vi "TCCII.vi"() -> ()   [LabVIEW 2019]
uses:
  <vilib>/Utility/NIReport.llb/Report Type.ctl
  <vilib>/Utility/NIReport.llb/image depth.ctl
  <vilib>/Instr/_visa.llb/VISA Configure Serial Port (Instr).vi
  <vilib>/Utility/NIReport.llb/Append Report Text (str wrap).vi
  <vilib>/printing/OpenHTMLReport.llb/Open HTML Report in Browser (Refnum).vi
  <vilib>/Utility/NIReport.llb/NI_report.lvclass
  <vilib>/Utility/NIReport.llb/NI_ReportGenerationCore.lvlib
panel:
  in  "ação":bool
  in  "Ação:":u16(ring) items=["Arquivo HTML", "Imprimir"]
  out "Temporary HTML file created 3":path
  out "grafico2":waveform(dbl)(graph) caption="Luminosidade"
  out "grafico1":waveform(dbl)[](graph) caption="Luminosidade"
  out "UV":u8(slide) scale=0.0..11.0
  out "INDICE UV":dbl
  out "INTENSIDADE":string
  out "TEMPERATURA":dbl(slide) scale=0.0..100.0
  out "UMIDADE":dbl(slide) scale=0.0..100.0
  out "LUMINOSIDADE":dbl(slide) scale=0.0..100.0
  out "Horário":timestamp format="%<%H:%M:%S\n%x>T"
  out "leitura":string
  out "Data 1D":dbl[](array[numeric])
  in  "Read count":u32
  in  "VISA Port":refnum<visa-resource-name>
  in  "Start reading":bool
  in  "parar":bool
  # "MONITORAMENTO PLANTA钦ES"
  # "INDICE UV"
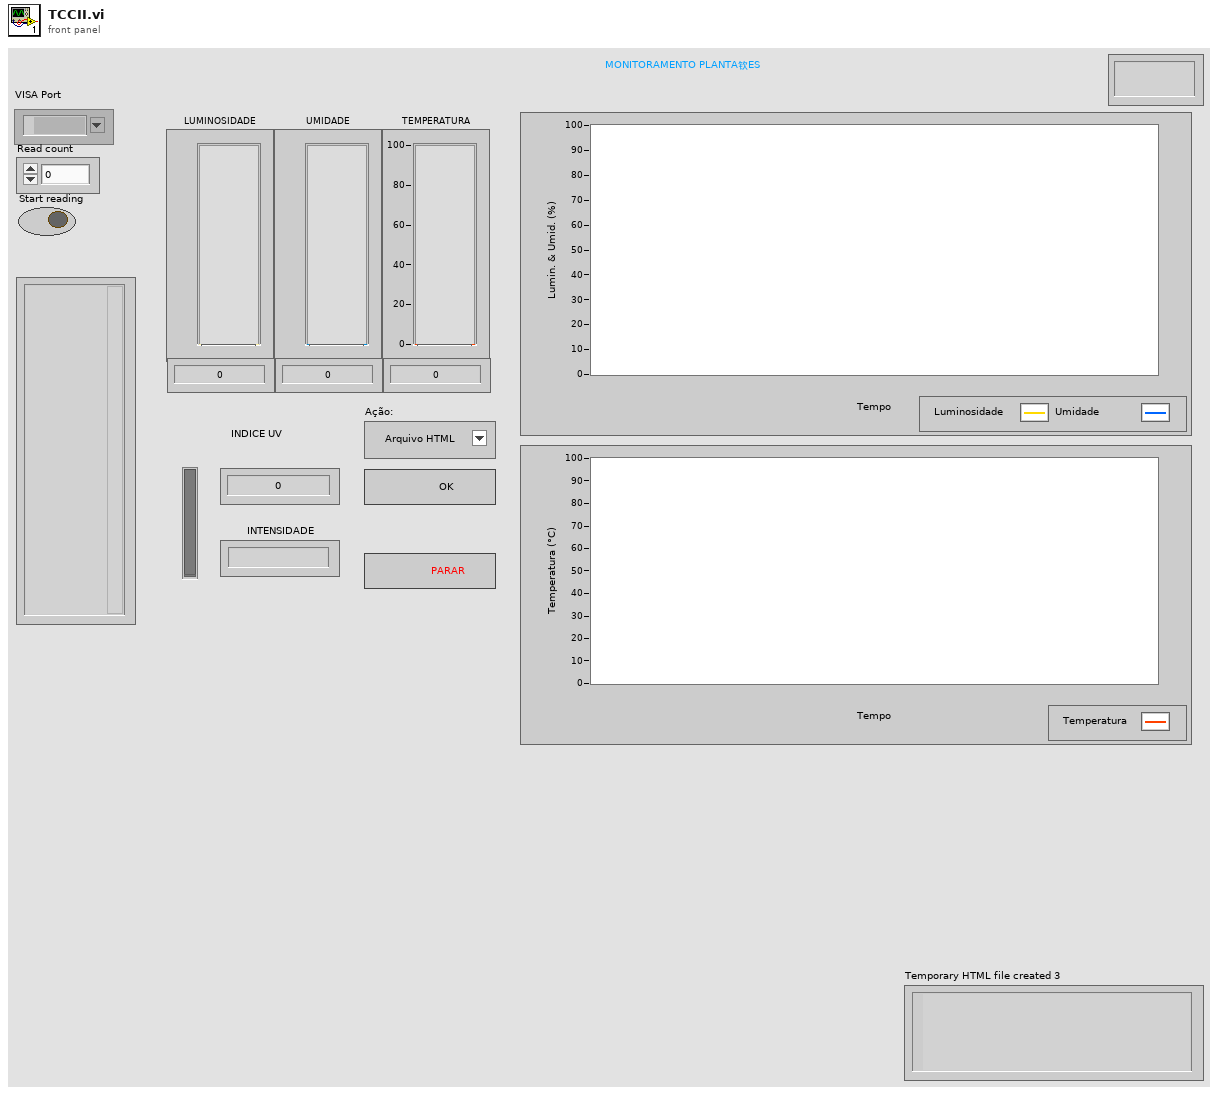
[diagram p1: front panel]
types:
  T1 = typedef "NI_ReportGenerationCore.lvlib/Report Type.ctl" = enum16{"HTML", "Word", "Excel"}
  T2 = typedef "NI_ReportGenerationCore.lvlib/image depth.ctl" = u16
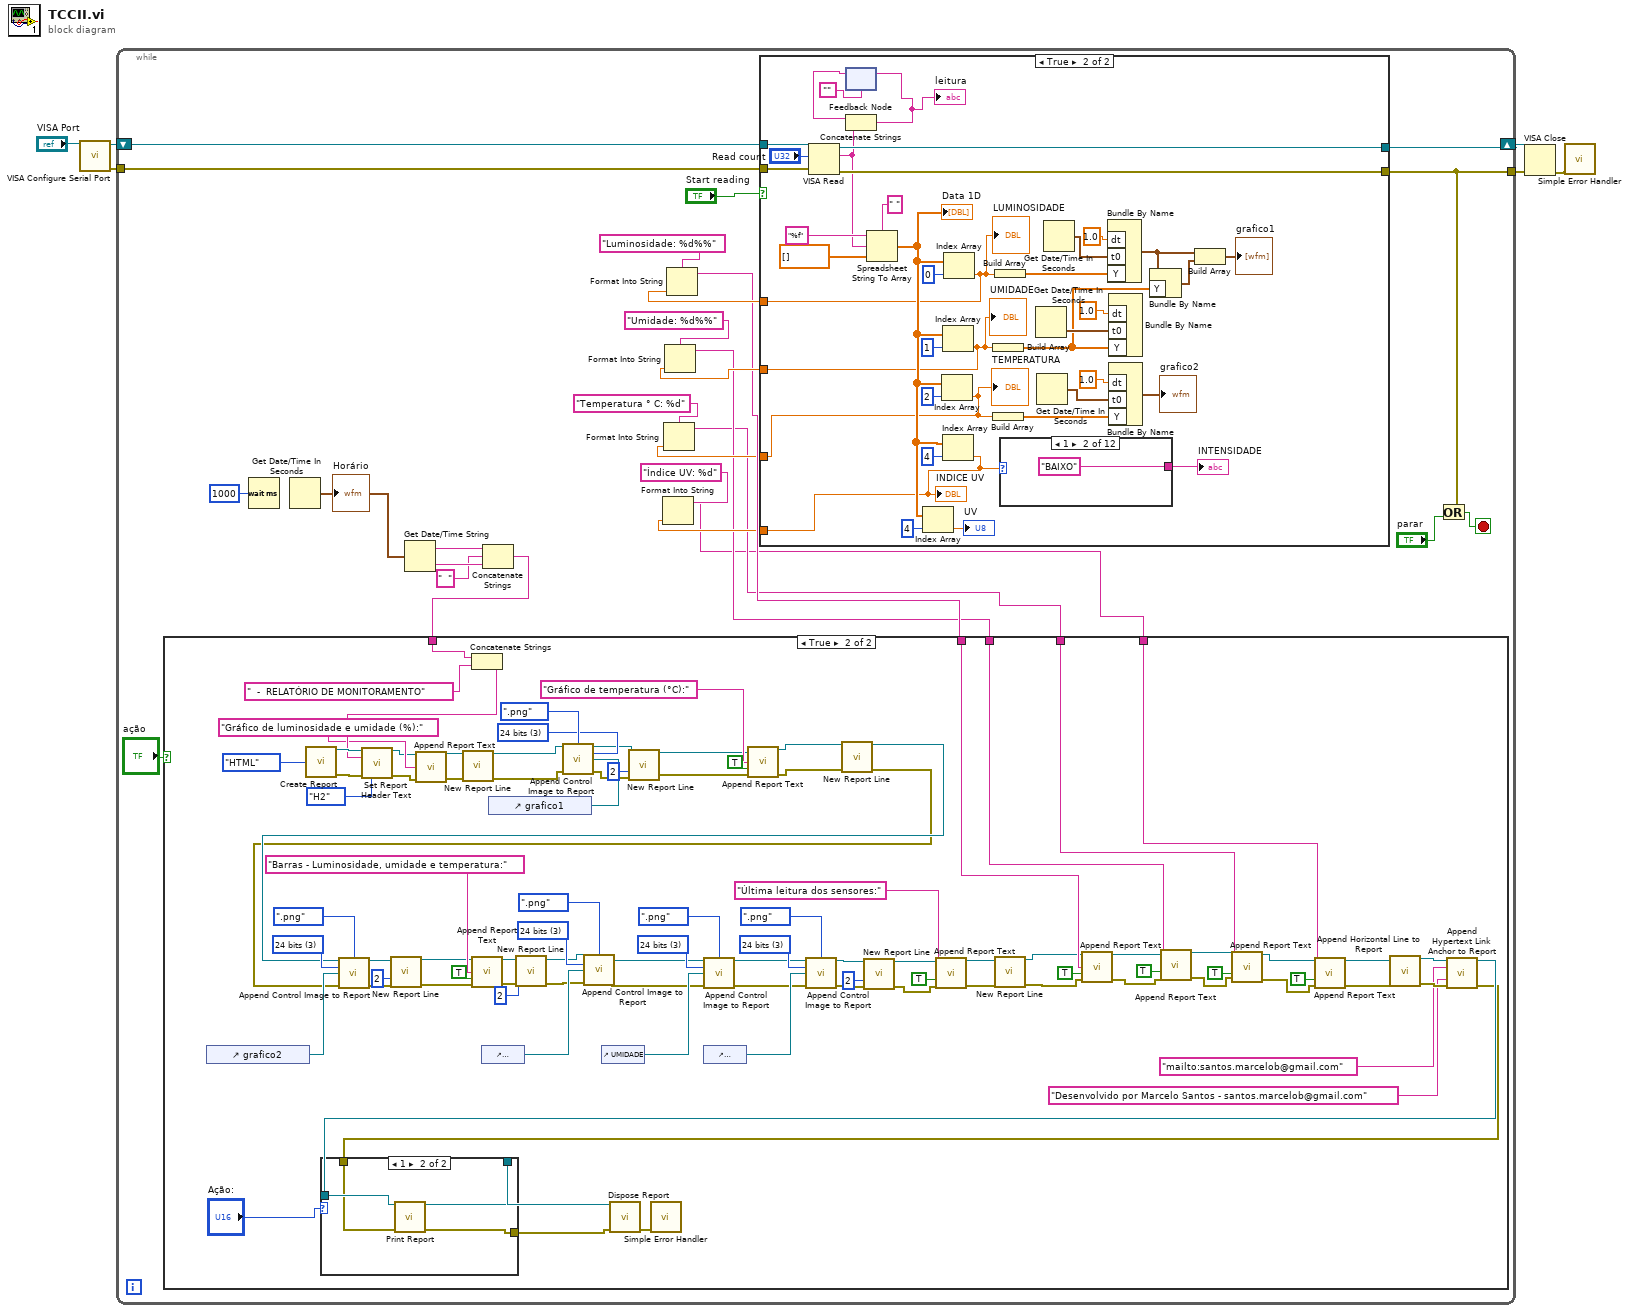
[diagram p0: block diagram]
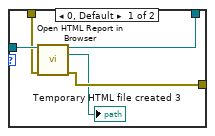
[diagram p3: hidden frame]
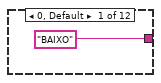
[diagram p5: hidden frame]
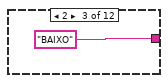
[diagram p6: hidden frame]
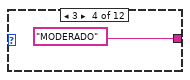
[diagram p7: hidden frame]
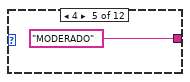
[diagram p8: hidden frame]
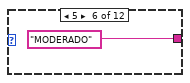
[diagram p9: hidden frame]
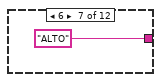
[diagram p10: hidden frame]
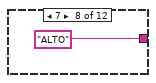
[diagram p11: hidden frame]
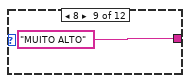
[diagram p12: hidden frame]
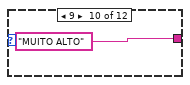
[diagram p13: hidden frame]
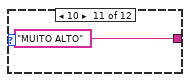
[diagram p14: hidden frame]
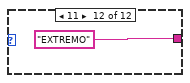
[diagram p15: hidden frame]
diagram:
  n1 = call-poly "VISA Configure Serial Port"("VISA resource name"="VISA Port") -> ("VISA resource name out"=w5:refnum<visa-resource-name>, "error out"=w2:errorcluster)  [unwired: 13 in]
  n2 = while {
    shift-right: [w29] -> w3
    shift-left: w5 -> [w30]
    tunnel: w2 -> [w28]
    tunnel: [w27] -> w1
    stop <- w26 stop-if-true
    n3 = Wait (ms)(milliseconds to wait=u32 1000) -> ()  [unwired: 1 out]
    n4 = Get Date/Time In Seconds() -> (seconds since 1Jan1904=w24:timestamp)
    "Horário" <- w24
    n5 = Get Date/Time String(seconds (now)=w24) -> (date string=w23:string, time string=w22:string)  [unwired: 2 in]
    n6 = Concatenate Strings(w23, "  " ("string"), w22) -> (w20:string)
    n7 = case shown="True" "Start reading" {
      tunnel: w30 -> [w136 w173]
      tunnel: [w136 w172] -> w29
      tunnel: w28 -> [w135 w170]
      tunnel: [w135 w169] -> w27
      tunnel: [_ w140] -> w16
      tunnel: [_ w139] -> w15
      tunnel: [_ w138] -> w12
      tunnel: [_ w137] -> w11
      frame False {
      }
      frame True {
        n8 = VISA Read(VISA resource name=w173, byte count="Read count", error in (no error)=w170) -> (VISA resource name out=w172:refnum<visa-resource-name>, read buffer=w165:string, error out=w169:errorcluster)  [unwired: 1 out]
        n9 = feedback #1("") -> (w164:string)
        n10 = Concatenate Strings(w164, w165) -> (w141:string)
        "leitura" <- w141
        n11 = feedback-in #1(w141) -> ()
        n12 = Spreadsheet String To Array(delimiter (Tab)=" ", format string="%f", spreadsheet string=w165, array type (2D Dbl)=dbl[] []) -> (array=w151:dbl[])
        "Data 1D" <- w151
        n13 = Index Array(array=w151, index=4) -> (element=→"UV":dbl)
        n14 = Index Array(array=w151, index=2) -> (element=w138:dbl)
        "TEMPERATURA" <- w138
        n15 = Index Array(array=w151, index=1) -> (element=w139:dbl)
        "UMIDADE" <- w139
        n16 = Index Array(array=w151, index=4) -> (element=w137:dbl)
        "INDICE UV" <- w137
        n17 = Index Array(array=w151, index=0) -> (element=w140:dbl)
        "LUMINOSIDADE" <- w140
        n18 = Build Array(w139) -> (w144:dbl[])
        n19 = Build Array(w138) -> (w145:dbl[])
        n20 = Build Array(w140) -> (w148:dbl[])
        n21 = case shown="1" w137 {
          tunnel: ["BAIXO" ("String") "BAIXO" ("String") "BAIXO" ("String") "MODERADO" ("String") "MODERADO" ("String") "MODERADO" ("String") "ALTO" ("String") "ALTO" ("String") "MUITO ALTO" ("String") "MUITO ALTO" ("String") "MUITO ALTO" ("String") "EXTREMO" ("String")] -> w153
          frame 0, Default {
          }
          frame 1 {
          }
          frame 2 {
          }
          frame 3 {
          }
          frame 4 {
          }
          frame 5 {
          }
          frame 6 {
          }
          frame 7 {
          }
          frame 8 {
          }
          frame 9 {
          }
          frame 10 {
          }
          frame 11 {
          }
        }
        "INTENSIDADE" <- w153
        n22 = Get Date/Time In Seconds() -> (seconds since 1Jan1904=w158:timestamp)
        n23 = Get Date/Time In Seconds() -> (seconds since 1Jan1904=w156:timestamp)
        n24 = Get Date/Time In Seconds() -> (seconds since 1Jan1904=w149:timestamp)
        n25 = Bundle By Name("dt"=1.0, "t0"=w149, "Y"=w148) -> (w143:waveform(dbl))  [unwired: 1 in]
        n26 = Bundle By Name("dt"=1.0, "t0"=w158, "Y"=w144) -> ()  [unwired: 1 in, 1 out]
        n27 = Bundle By Name("dt"=1.0, "t0"=w156, "Y"=w145) -> (→"grafico2":waveform(dbl))  [unwired: 1 in]
        n28 = Bundle By Name(cluster=w143, "Y"=w144) -> (w146:waveform(dbl))
        n29 = Build Array(w143, w146) -> (→"grafico1":waveform(dbl)[])
      }
    }
    n30 = Format Into String(format string="Índice UV: %d", w11) -> (resulting string=w8:string)  [unwired: 2 in, 1 out]
    n31 = Format Into String(format string="Temperatura ° C: %d", w12) -> (resulting string=w9:string)  [unwired: 2 in, 1 out]
    n32 = Format Into String(format string="Umidade: %d%%", w15) -> (resulting string=w10:string)  [unwired: 2 in, 1 out]
    n33 = Format Into String(format string="Luminosidade: %d%%", w16) -> (resulting string=w14:string)  [unwired: 2 in, 1 out]
    n34 = case shown="True" "ação" {
      tunnel: w20 -> [_ w110]
      tunnel: w14 -> [_ w79]
      tunnel: w10 -> [_ w75]
      tunnel: w9 -> [_ w74]
      tunnel: w8 -> [_ w73]
      frame False {
      }
      frame True {
        w100 = T2 3 items=["B&W", "4 bits", "8 bits", "24 bits"] ("image depth")
        w101 = T2 3 items=["B&W", "4 bits", "8 bits", "24 bits"] ("image depth")
        w106 = T2 3 items=["B&W", "4 bits", "8 bits", "24 bits"] ("image depth")
        w113 = T2 3 items=["B&W", "4 bits", "8 bits", "24 bits"] ("image depth")
        w118 = T2 3 items=["B&W", "4 bits", "8 bits", "24 bits"] ("image depth")
        n35 = control-ref of="grafico2"() -> (w115:refnum<vi>)
        n36 = call <vilib>:"Create Report.vi"("report type"=Report_Type."HTML" ("Report Type")) -> ("report out"=w124:refnum<class "NI_report.lvclass">, "error out"=w125:errorcluster)  [unwired: 13 in]
        n37 = Concatenate Strings(w110, "  -  RELATÓRIO DE MONITORAMENTO" ("string")) -> (w108:string)
        n38 = call-dynamic "Set Report Header Text.vi"("report in"=w124, "left header text"=w108, "error in (no error)"=w125, "HTML header size"=enum16{"H1", "H2", "H3", "H4", "H5", "H6", "H7"}."H2") -> ("report out"=w39:refnum<class "NI_report.lvclass">, "error out"=w38:errorcluster)  [unwired: 10 in]
        n39 = call-poly <vilib>:"Append Report Text.vi"("report in"=w39, "text"="Gráfico de luminosidade e umidade (%):", "error in (no error)"=w38) -> ("report out"=w35:refnum<class "NI_report.lvclass">, "error out"=w36:errorcluster)  [unwired: 9 in, 2 out]
        n40 = call-dynamic "New Report Line.vi"("report in"=w35, "error in (no error)"=w36) -> ("report out"=w34:refnum<class "NI_report.lvclass">, "error out"=w37:errorcluster)  [unwired: 12 in]
        n41 = control-ref of="LUMINOSIDADE"() -> (w104:refnum<vi>)
        n42 = control-ref of="grafico1"() -> (w121:refnum<vi>)
        n43 = call-dynamic "Append Control Image to Report.vi"("report in"=w34, "image file type (.jpg)"=enum16{".jpg", ".png"}.".png" ("image file type"), "image depth"=w118, "ctrl reference"=w121, "error in (no error)"=w37) -> ("report out"=w54:refnum<class "NI_report.lvclass">, "error out"=w55:errorcluster)  [unwired: 7 in, 2 out]
        n44 = control-ref of="UMIDADE"() -> (w103:refnum<vi>)
        n45 = call-dynamic "New Report Line.vi"("report in"=w54, "number of lines (1)"=2, "error in (no error)"=w55) -> ("report out"=w57:refnum<class "NI_report.lvclass">, "error out"=w56:errorcluster)  [unwired: 11 in]
        n46 = control-ref of="TEMPERATURA"() -> (w98:refnum<vi>)
        n47 = call-poly <vilib>:"Append Report Text.vi"("report in"=w57, "text"="Gráfico de temperatura (°C):", "append on new line? (F)"=TRUE, "error in (no error)"=w56) -> ("report out"=w42:refnum<class "NI_report.lvclass">, "error out"=w43:errorcluster)  [unwired: 8 in, 2 out]
        n48 = call-dynamic "New Report Line.vi"("report in"=w42, "error in (no error)"=w43) -> ("report out"=w41:refnum<class "NI_report.lvclass">, "error out"=w40:errorcluster)  [unwired: 12 in]
        n49 = call-dynamic "Append Control Image to Report.vi"("report in"=w41, "image file type (.jpg)"=enum16{".jpg", ".png"}.".png", "image depth"=w113, "ctrl reference"=w115, "error in (no error)"=w40) -> ("report out"=w51:refnum<class "NI_report.lvclass">, "error out"=w52:errorcluster)  [unwired: 7 in, 2 out]
        n50 = call-dynamic "New Report Line.vi"("report in"=w51, "number of lines (1)"=2, "error in (no error)"=w52) -> ("report out"=w50:refnum<class "NI_report.lvclass">, "error out"=w49:errorcluster)  [unwired: 11 in]
        n51 = call-poly <vilib>:"Append Report Text.vi"("report in"=w50, "text"="Barras - Luminosidade, umidade e temperatura:", "append on new line? (F)"=TRUE, "error in (no error)"=w49) -> ("report out"=w96:refnum<class "NI_report.lvclass">, "error out"=w97:errorcluster)  [unwired: 8 in, 2 out]
        n52 = call-dynamic "New Report Line.vi"("report in"=w96, "number of lines (1)"=2, "error in (no error)"=w97) -> ("report out"=w93:refnum<class "NI_report.lvclass">, "error out"=w92:errorcluster)  [unwired: 11 in]
        n53 = call-dynamic "Append Control Image to Report.vi"("report in"=w93, "image file type (.jpg)"=enum16{".jpg", ".png"}.".png", "image depth"=w106, "ctrl reference"=w104, "error in (no error)"=w92) -> ("report out"=w90:refnum<class "NI_report.lvclass">, "error out"=w91:errorcluster)  [unwired: 7 in, 2 out]
        n54 = call-dynamic "Append Control Image to Report.vi"("report in"=w90, "image file type (.jpg)"=enum16{".jpg", ".png"}.".png", "image depth"=w101, "ctrl reference"=w103, "error in (no error)"=w91) -> ("report out"=w89:refnum<class "NI_report.lvclass">, "error out"=w88:errorcluster)  [unwired: 7 in, 2 out]
        n55 = call-dynamic "Append Control Image to Report.vi"("report in"=w89, "image file type (.jpg)"=enum16{".jpg", ".png"}.".png", "image depth"=w100, "ctrl reference"=w98, "error in (no error)"=w88) -> ("report out"=w65:refnum<class "NI_report.lvclass">, "error out"=w66:errorcluster)  [unwired: 7 in, 2 out]
        n56 = call-dynamic "New Report Line.vi"("report in"=w65, "number of lines (1)"=2, "error in (no error)"=w66) -> ("report out"=w62:refnum<class "NI_report.lvclass">, "error out"=w61:errorcluster)  [unwired: 11 in]
        n57 = call-poly <vilib>:"Append Report Text.vi"("report in"=w62, "text"="Última leitura dos sensores:", "append on new line? (F)"=TRUE, "error in (no error)"=w61) -> ("report out"=w46:refnum<class "NI_report.lvclass">, "error out"=w47:errorcluster)  [unwired: 8 in, 2 out]
        n58 = call-dynamic "New Report Line.vi"("report in"=w46, "error in (no error)"=w47) -> ("report out"=w45:refnum<class "NI_report.lvclass">, "error out"=w44:errorcluster)  [unwired: 12 in]
        n59 = call-poly <vilib>:"Append Report Text.vi"("report in"=w45, "text"=w79, "append on new line? (F)"=TRUE, "error in (no error)"=w44) -> ("report out"=w72:refnum<class "NI_report.lvclass">, "error out"=w71:errorcluster)  [unwired: 8 in, 2 out]
        n60 = call-poly <vilib>:"Append Report Text.vi"("report in"=w72, "text"=w75, "append on new line? (F)"=TRUE, "error in (no error)"=w71) -> ("report out"=w69:refnum<class "NI_report.lvclass">, "error out"=w70:errorcluster)  [unwired: 8 in, 2 out]
        n61 = call-poly <vilib>:"Append Report Text.vi"("report in"=w69, "text"=w74, "append on new line? (F)"=TRUE, "error in (no error)"=w70) -> ("report out"=w68:refnum<class "NI_report.lvclass">, "error out"=w67:errorcluster)  [unwired: 8 in, 2 out]
        n62 = call-poly <vilib>:"Append Report Text.vi"("report in"=w68, "text"=w73, "append on new line? (F)"=TRUE, "error in (no error)"=w67) -> ("report out"=w58:refnum<class "NI_report.lvclass">, "error out"=w33:errorcluster)  [unwired: 8 in, 2 out]
        n63 = call-dynamic "Append Horizontal Line to Report.vi"("report in"=w58, "error in (no error)"=w33) -> ("report out"=w120:refnum<class "NI_report.lvclass">, "error out"=w119:errorcluster)  [unwired: 12 in]
        n64 = call-dynamic "Append Hypertext Link Anchor to Report.vi"("report in"=w120, "URL of link - href"="mailto:santos.marcelob@gmail.com", "link text"="Desenvolvido por Marcelo Santos - santos.marcelob@gmail.com", "error in (no error)"=w119) -> ("report out"=w86:refnum<class "NI_report.lvclass">, "error out"=w85:errorcluster)  [unwired: 8 in, 2 out]
        n65 = case shown="1" "Ação:" {
          tunnel: w86 -> [w130 w132]
          tunnel: w85 -> [w129 w131]
          tunnel: [w128 w134] -> w84
          tunnel: [w127 w133] -> w83
          frame 0, Default {
            n66 = call-poly <vilib>:"Open HTML Report in Browser.vi"("report in"=w130, "error in (no error)"=w129) -> ("report out"=w128:refnum<class "NI_report.lvclass">, "temporary HTML file created"=→"Temporary HTML file created 3":path, "error out"=w127:errorcluster)  [unwired: 11 in]
          }
          frame 1 {
            n67 = call-dynamic "Print Report.vi"("report in"=w132, "error in (no error)"=w131) -> ("report out"=w134:refnum<class "NI_report.lvclass">, "error out"=w133:errorcluster)  [unwired: 12 in]
          }
        }
        n68 = call-dynamic "Dispose Report.vi"("report in"=w84, "error in (no error)"=w83) -> ("error out"=w116:errorcluster)  [unwired: 13 in]
        n69 = call <vilib>:"Simple Error Handler.vi"("error in (no error)"=w116) -> ()  [unwired: 4 in, 5 out]
      }
    }
    n70 = Or(x=w27, y="parar") -> (x .or. y?=w26:bool)
  }
  n71 = VISA Close(VISA resource name=w3, error in (no error)=w1) -> (error out=w4:errorcluster)
  n72 = call <vilib>:"Simple Error Handler.vi"("error in (no error)"=w4) -> ()  [unwired: 4 in, 5 out]
